vi "Sensor2String.vi"(8 "error in (no error)":errorcluster, 11 "Sensor DAO Class in":refnum<class "Sensor DAO Class.lvclass">) -> (0 "error out":errorcluster, 2 "Strings":string[](array[string]), 3 "Sensor DAO Class out":refnum<class "Sensor DAO Class.lvclass">)   [LabVIEW 2013, in "Sensor DAO Class.lvclass"]
uses:
  Sensor DAO Class.lvclass
  Sensor DAO Class.lvclass/Sensor DAO Class.ctl
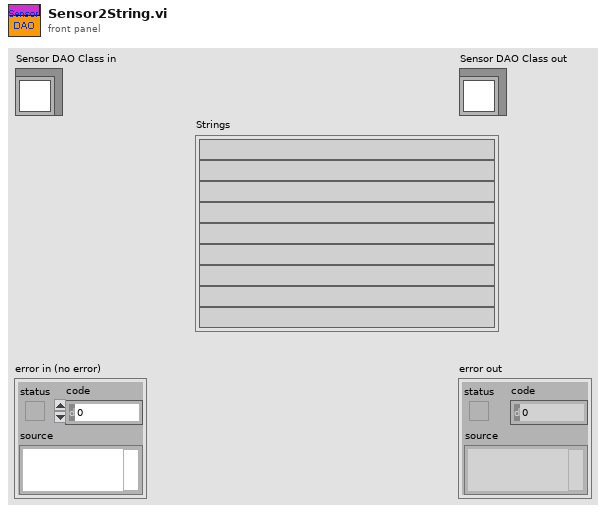
[diagram p1: front panel]
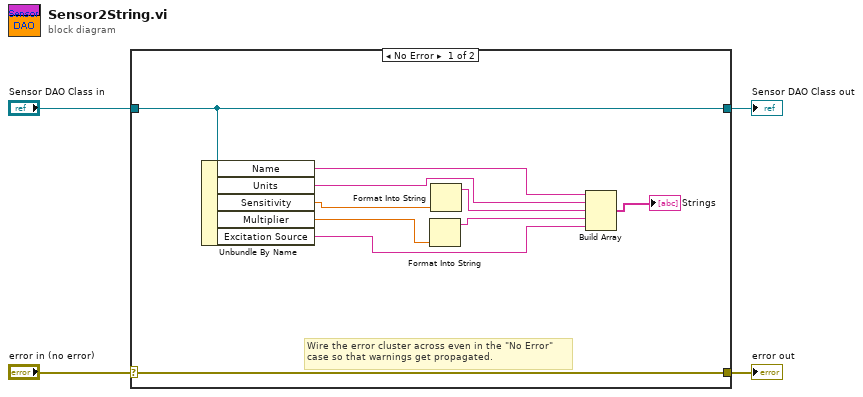
[diagram p0: block diagram]
diagram:
  n1 = case shown="No Error" "error in (no error)" {
    selector: "error in (no error)" -> [w14 w16]
    tunnel: [w14 w16] -> w3
    tunnel: [w13 w15] -> w1
    tunnel: "Sensor DAO Class in" -> [w13 w15]
    frame No Error {
      # "Wire the error cluster across even in the \"No Error\"\ncase so that warnings get propagated."
      n2 = Unbundle By Name(w13) -> ("Name"=w12:string, "Units"=w11:string, "Sensitivity"=w10:dbl, "Multiplier"=w8:dbl, "Excitation Source"=w6:string)
      n3 = Format Into String(w8) -> (resulting string=w7:string)  [unwired: 3 in, 1 out]
      n4 = Format Into String(w10) -> (resulting string=w9:string)  [unwired: 3 in, 1 out]
      n5 = Build Array(w12, w11, w9, w7, w6) -> (→"Strings":string[])
    }
    frame Error {
    }
  }
  "error out" <- w3
  "Sensor DAO Class out" <- w1
